vi "SH_displayResults.vi"(2 "Control Refs":T1, 4 "Shapelet Notifier":refnum<notifier>) -> ()   [LabVIEW 2016, in "Shapelets Search (Brute Force).lvlib"]
uses:
  Shapelets Search (Brute Force).lvlib
  SH_Shapelet.ctl
panel:
  # "This VI is a part of BCI Design library, http://www.ru-bci.org \nCopyright © 2020, Sotnikov Peter, All rights reserved. License: CC BY-NC 4.0"
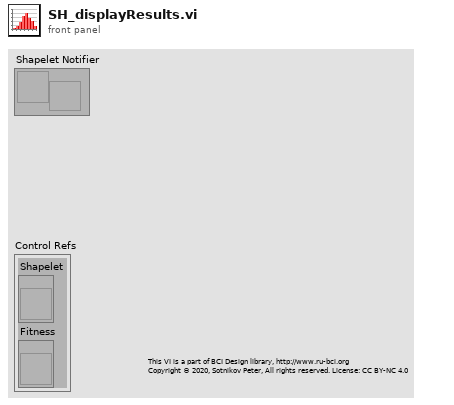
[diagram p1: front panel]
types:
  T1 = cluster{"Shapelet":refnum<vi>, "Fitness":refnum<vi>}
  T2 = typedef "Shapelets Search (Brute Force).lvlib/SH_Shapelet.ctl" = cluster{"TrialIndex":i32, "Shift (in samples)":i32, "Length (in samples)":i32, "Distances":dbl[], "ClassIndecies":i32[], "Fitness":dbl, "Split Point":dbl}
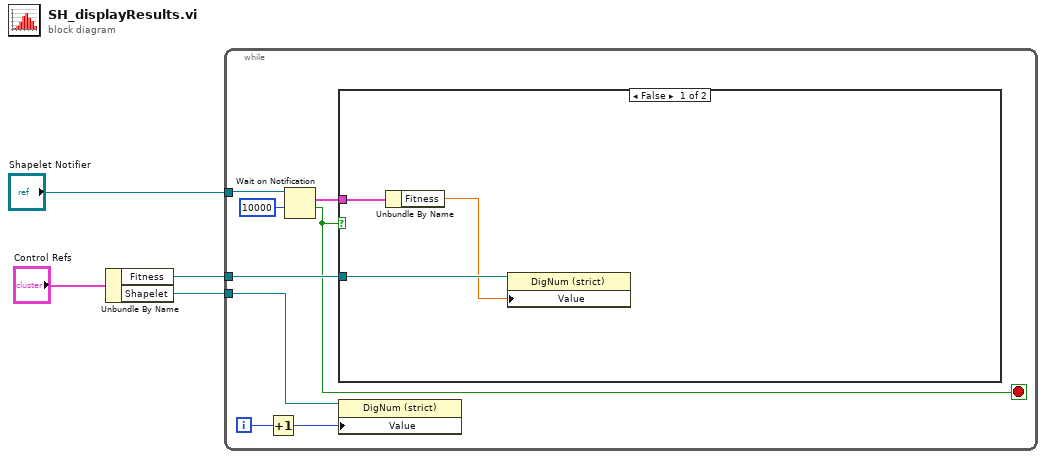
[diagram p0: block diagram]
diagram:
  n1 = Unbundle By Name("Control Refs") -> ("Fitness"=w2:refnum<vi>, "Shapelet"=w1:refnum<vi>)
  n2 = while {
    tunnel: "Shapelet Notifier" -> [w12]
    tunnel: w2 -> [w6]
    tunnel: w1 -> [w8]
    i -> [w11]
    stop <- w5 stop-if-true
    n3 = Increment(x=w11) -> (x+1=w7:i32)
    n4 = Wait on Notification(notifier=w12, timeout in ms (-1)=10000) -> (notification=w10:T2, timed out?=w5:bool)  [unwired: 2 in, 2 out]
    n5 = case shown="False" w5 {
      tunnel: w10 -> [w15 _]
      tunnel: w6 -> [w14 _]
      frame False {
        n6 = Unbundle By Name(w15) -> ("Fitness"=w13:dbl)
        n7 = property class="DigNum (strict)"(reference=w14, "Value"=w13) -> ()  [unwired: 1 in, 2 out]
      }
      frame True {
      }
    }
    n8 = property class="DigNum (strict)"(reference=w8, "Value"=w7) -> ()  [unwired: 1 in, 2 out]
  }
